vi "DrawSubMenu.vi"(7 "Tag":string, 8 "error in (no error)":errorcluster, 9 "Pict Refnum":refnum<vi>, 10 "Coords":T2, 11 "Menu in":refnum<class "Menu.lvclass">) -> (0 "error out":errorcluster, 1 "Global Area":T1, 2 "Selected Area":T1, 3 "Menu out":refnum<class "Menu.lvclass">, 4 "SubMenu":bool, 5 "Selected Tag":string)   [LabVIEW 2021, in "Menu.lvlib" / "Menu.lvclass"]
uses:
  Menu.lvclass
  Menu.lvclass/Menu.ctl
  Picture2D/src/Collection/Collection.lvclass
  Picture2D/src/2DPictureControl/2DPictureControl.lvclass
  C:/GitHub/Picture2D/src/Picture2D/Picture2D.lvclass
  C:/GitHub/Picture2D/src/IDrawable/IDrawable.lvclass
  C:/GitHub/Picture2D/src/IMovable/IMovable.lvclass
  C:/GitHub/Picture2D/src/IRotatable/IRotatable.lvclass
  C:/GitHub/Picture2D/src/IScalable/IScalable.lvclass
  C:/GitHub/Picture2D/src/Collection/Collection.lvclass
  <vilib>/Utility/miscctls.llb/LVPoint32TypeDef.ctl
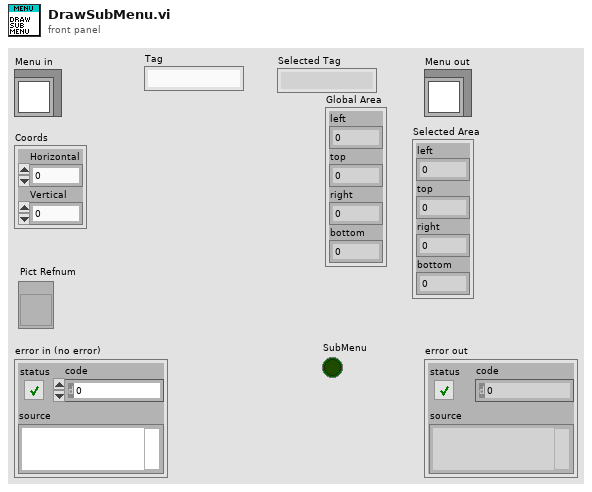
[diagram p1: front panel]
types:
  T1 = cluster{"left":i16, "top":i16, "right":i16, "bottom":i16}
  T2 = typedef "LVPoint32TypeDef.ctl" = cluster{"Horizontal":i32, "Vertical":i32}
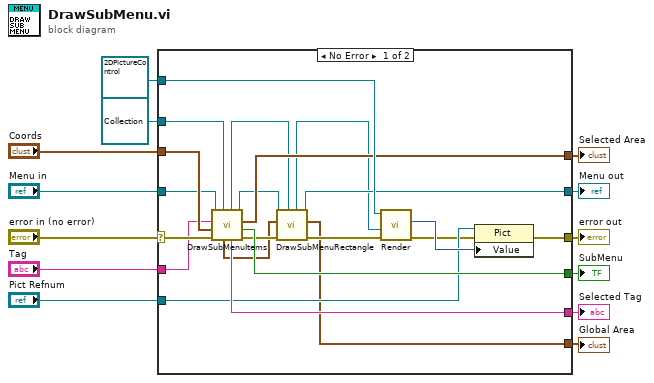
[diagram p0: block diagram]
diagram:
  n1 = case shown="No Error" "error in (no error)" {
    selector: "error in (no error)" -> [w27 w35]
    tunnel: [w33 _] -> w13
    tunnel: [w21 _] -> w12
    tunnel: [w32 w35] -> w11
    tunnel: [w31 _] -> w10
    tunnel: "Coords" -> [w29 _]
    tunnel: [w18 w36] -> w7
    tunnel: "Menu in" -> [w25 w36]
    tunnel: refnum<class "Collection.lvclass"> refnum ("Picture2D.lvlib:Collection.lvclass") -> [w26 _]
    tunnel: refnum<class "2DPictureControl.lvclass"> refnum ("2DPictureControl in") -> [w28 _]
    tunnel: "Pict Refnum" -> [w24 _]
    tunnel: "Tag" -> [w22 _]
    tunnel: [w16 _] -> w1
    frame No Error {
      n2 = call "DrawSubMenuItems.vi"("Collection in"=w26, "error in (no error)"=w27, "Coords"=w29, "Tag"=w22, "Menu in"=w25) -> ("error out"=w30:errorcluster, "SubMenu"=w31:bool, "SelectedArea"=w21:T1, "Menu out"=w19:refnum<class "Menu.lvclass">, "SelectedItemTag"=w33:string, "Collection out"=w15:refnum<class "Collection.lvclass">, "GlobalArea"=w17:T1)
      n3 = call "DrawSubMenuRectangle.vi"("Collection in"=w15, "error in (no error)"=w30, "Area"=w17, "Menu in"=w19) -> ("error out"=w20:errorcluster, "Area"=w16:T1, "Menu out"=w18:refnum<class "Menu.lvclass">, "Collection out"=w14:refnum<class "Collection.lvclass">)  [unwired: 4 in]
      n4 = call-dynamic "Render.vi"("error in (no error)"=w20, "IDrawable"=w14, "2DPictureControl in"=w28) -> ("error out"=w23:errorcluster, "2D Picture out"=w34:picture)  [unwired: 6 in, 1 out]
      n5 = property class="Pict"(reference=w24, error in=w23, "Value"=w34) -> (error out=w32:errorcluster)  [unwired: 1 out]
    }
    frame Error {
    }
  }
  "Selected Tag" <- w13
  "Selected Area" <- w12
  "error out" <- w11
  "Menu out" <- w7
  "SubMenu" <- w10
  "Global Area" <- w1
